vi "GetRtd9226Properties.vi"(11 "Properties":T1[](array[typedef])) -> (0 "B":dbl, 1 "A":dbl, 2 "RTD type":u32, 3 "RTD ohm degree range":u32, 4 "C":dbl, 6 "r0":dbl)   [LabVIEW 2017, in "ScanEngine.lvlib"]
uses:
  <vilib>/addons/InsightCM/Devices/Shared/Common/ScanEngine/ScanEngine.lvlib
  <vilib>/addons/InsightCM/MessageBus/Base/controls/KeyValuePair.ctl
  <vilib>/Utility/miscctls.llb/LVStringsAndValuesArrayTypeDef_U32.ctl
  <vilib>/addons/InsightCM/Utilities/PropertyHelpers/PropertyHelpers.lvlib
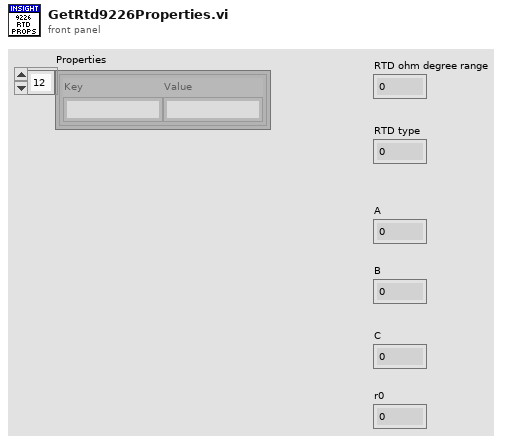
[diagram p1: front panel]
types:
  T1 = typedef "KeyValuePair.ctl" = cluster{"Key":string, "Value":string}
  T2 = typedef "LVStringsAndValuesArrayTypeDef_U32.ctl" = cluster{"String":string, "Value":u32}[]
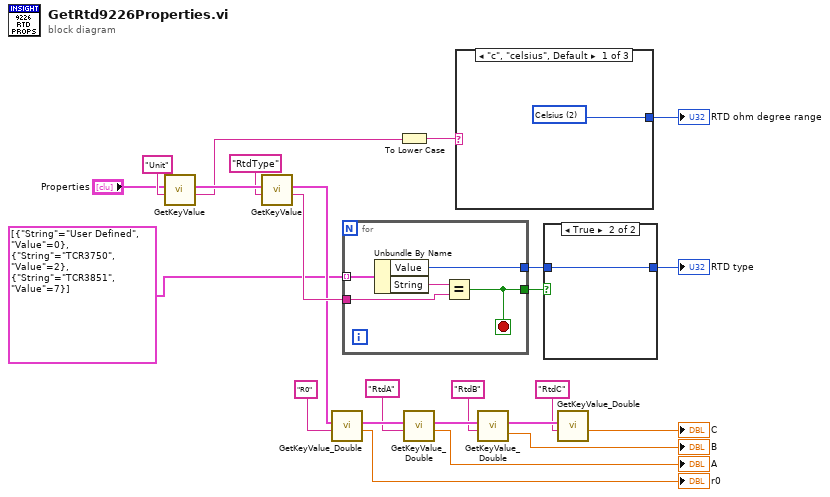
[diagram p0: block diagram]
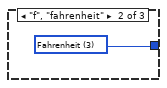
[diagram p2: hidden frame]
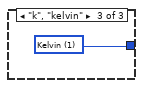
[diagram p3: hidden frame]
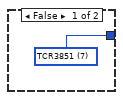
[diagram p4: hidden frame]
diagram:
  n1 = call <vilib>:"GetKeyValue.vi"("key"="Unit" ("name"), "key value pairs"="Properties") -> ("value"=w4:string, "key value pairs out"=w11:T1[])  [unwired: 7 in, 1 out]
  n2 = call <vilib>:"GetKeyValue.vi"("key"="RtdType" ("name"), "key value pairs"=w11) -> ("value"=w8:string, "key value pairs out"=w5:T1[])  [unwired: 7 in, 1 out]
  n3 = call <vilib>:"GetKeyValue_Double.vi"("key"="R0" ("name"), "key value pairs"=w5) -> ("value"=→"r0":dbl, "key value pairs out"=w24:T1[])  [unwired: 7 in, 1 out]
  n4 = for {
    tunnel: T2 [{"String"="User Defined", "Value"=0}, {"String"="TCR3750", "Value"=2}, {"String"="TCR3851", "Value"=7}] ("Strings And Values []") -> [w29] mode=indexing
    tunnel: [w27] -> w13
    tunnel: w8 -> [w26]
    tunnel: [w25] -> w12
    stop <- w25 stop-if-true
    n5 = Unbundle By Name(w29) -> ("Value"=w27:u32, "String"=w28:string)
    n6 = Equal?(x=w28, y=w26) -> (x = y?=w25:bool)
  }
  n7 = To Lower Case(string=w4) -> (all lower case string=w2:string)
  n8 = call <vilib>:"GetKeyValue_Double.vi"("key"="RtdA" ("name"), "key value pairs"=w24) -> ("value"=→"A":dbl, "key value pairs out"=w23:T1[])  [unwired: 7 in, 1 out]
  n9 = case shown="\"c\", \"celsius\", Default" w2 {
    tunnel: [w30 w31 w32] -> w3
    frame "c", "celsius", Default {
      w30 = u32 2 items=["Ohms", "Kelvin", "Celsius", "Fahrenheit", "Rankine"] ("RTD0:Ohm degree range")
    }
    frame "f", "fahrenheit" {
      w31 = u32 3 items=["Volts", "Kelvin", "Celsius", "Fahrenheit", "Rankine"] ("CH3:Degree range")
    }
    frame "k", "kelvin" {
      w32 = u32 1 items=["Volts", "Kelvin", "Celsius", "Fahrenheit", "Rankine"] ("CH3:Degree range")
    }
  }
  "RTD ohm degree range" <- w3
  n10 = call <vilib>:"GetKeyValue_Double.vi"("key"="RtdB" ("name"), "key value pairs"=w23) -> ("value"=→"B":dbl, "key value pairs out"=w22:T1[])  [unwired: 7 in, 1 out]
  n11 = case shown="True" w12 {
    tunnel: [w33 w34] -> w6
    tunnel: w13 -> [_ w34]
    frame False {
      w33 = u32 7 items=["User Defined"=0, "TCR3750"=2, "TCR3851"=7] ("RTD0:RTD type")
    }
    frame True {
    }
  }
  "RTD type" <- w6
  n12 = call <vilib>:"GetKeyValue_Double.vi"("key"="RtdC" ("name"), "key value pairs"=w22) -> ("value"=→"C":dbl)  [unwired: 7 in, 2 out]
